vi "Flatten.vi"(6 "FIFO Timestamps":T1, 8 "error in (no error)":errorcluster, 10 "Data in":u8[](array[numeric]) format="%.0x", 11 "CIFTag in":refnum<class "CIF_NIChn_FifoCAN.lvclass">) -> (0 "error out":errorcluster, 3 "CIFTag out":refnum<class "CIF_NIChn_FifoCAN.lvclass">)   [LabVIEW 2021, in "CIF_NIChn_FifoCAN.lvclass"]
uses:
  CIF_NIChn_FifoCAN.lvclass
  ChannelCommon/typedef/TimeStamps.ctl
  CIF_NIChn_FifoCAN.lvclass/CIF_NIChn_FifoCAN.ctl
  ChannelCommon/CIFFIFO/CIFfifo.lvclass/CIFfifo.ctl
  ChannelCommon/CIFFIFO/Accessors/Write T0.vi
  ChannelCommon/CIFFIFO/Accessors/Write T_Out.vi
  ChannelCommon/CIFFIFO/Accessors/Write ClockID.vi
  <vilib>/CIF Foundation/CIF Utilities/Time/System Time/Get System Time.vi
  ChannelCommon/Utilities/Flatten Header.vi
  ChannelCommon/CIFFIFO/Accessors/Write Payload Length.vi
  ChannelCommon/CIFFIFO/Accessors/Read Header.vi
  <vilib>/CIF Foundation/CIF Utilities/Time/System Time/LabVIEW Time to TAI Time.vi
  <vilib>/CIF Foundation/CIF Utilities/DataTypes/Flatten U64.vi
  <vilib>/CIF Foundation/CIF Utilities/DataTypes/Flatten I64.vi
  ChannelCommon/CIFFIFO/CIFfifo.lvclass
  ChannelCommon/ChannelCommon.lvlib
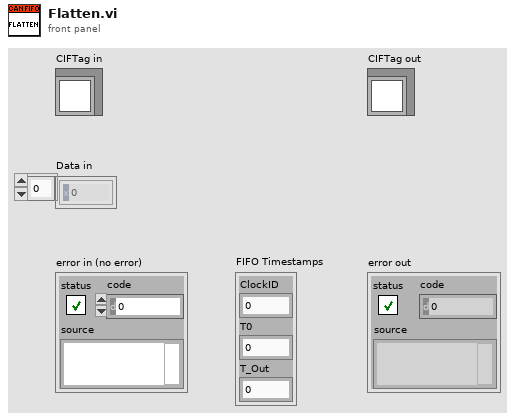
[diagram p1: front panel]
types:
  T1 = typedef "ChannelCommon.lvlib/TimeStamps.ctl" = cluster{"ClockID":u8, "T0":i64, "T_Out":i64}
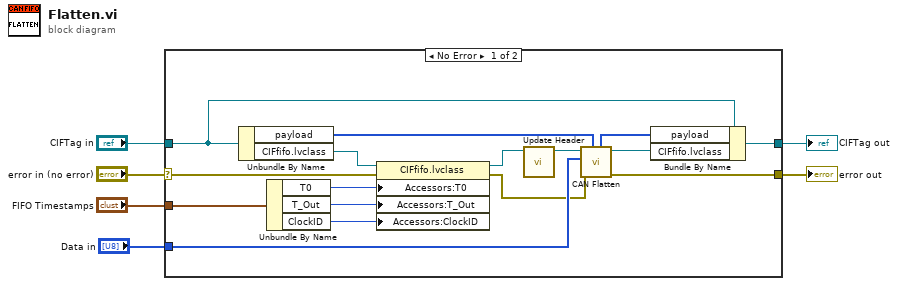
[diagram p0: block diagram]
diagram:
  n1 = case shown="No Error" "error in (no error)" {
    selector: "error in (no error)" -> [w20 w24]
    tunnel: [w22 w24] -> w5
    tunnel: [w21 w23] -> w3
    tunnel: "CIFTag in" -> [w19 w23]
    tunnel: "FIFO Timestamps" -> [w18 _]
    tunnel: "Data in" -> [w17 _]
    frame No Error {
      n2 = Unbundle By Name(w19) -> ("payload"=w13:u8[], "CIFfifo.lvclass"=w16:refnum<class "CIFfifo.lvclass">)
      n3 = Unbundle By Name(w18) -> ("T0"=w8:i64, "T_Out"=w9:i64, "ClockID"=w10:u8)
      n4 = property class="CIFfifo.lvclass"(reference=w16, error in=w20, "Accessors:T0"=w8, "Accessors:T_Out"=w9, "Accessors:ClockID"=w10) -> (reference out=w15:refnum<class "CIFfifo.lvclass">, error out=w7:errorcluster)
      n5 = call "Update Header.vi"("CIFFIFO in"=w15) -> ("CIFFIFO out"=w14:refnum<class "CIFfifo.lvclass">)  [unwired: 10 in]
      n6 = call "CAN Flatten.vi"("payload in"=w13, "error in (no error)"=w7, "Data in"=w17, "CIFFifo in"=w14) -> ("error out"=w22:errorcluster, "CIFFifo out"=w11:refnum<class "CIFfifo.lvclass">, "payload out"=w12:u8[])  [unwired: 5 in]
      n7 = Bundle By Name(cluster=w19, "payload"=w12, "CIFfifo.lvclass"=w11) -> (w21:refnum<class "CIF_NIChn_FifoCAN.lvclass">)
    }
    frame Error {
    }
  }
  "error out" <- w5
  "CIFTag out" <- w3
